vi "Object_number.vi"(1 "Insect-data-array":dbl[][](array[numeric])) -> (0 "Number of objects":i32)   [LabVIEW 2022 SP3]
doc: "Number of objects in the insect-data-array"
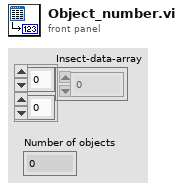
[diagram p1: front panel]
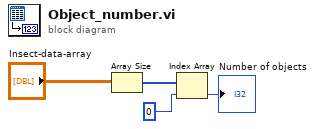
[diagram p0: block diagram]
diagram:
  n1 = Array Size(array="Insect-data-array") -> (size(s)=w2:i32[])
  n2 = Index Array(array=w2, index=0) -> (element=→"Number of objects":i32)
